vi "Reward Demo (SubVI).vi"(10 "Action":i32, 11 "State":i32) -> (3 "Reward":dbl format="%#_13g")   [LabVIEW 2013]
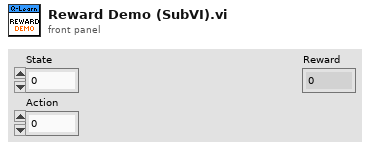
[diagram p1: front panel]
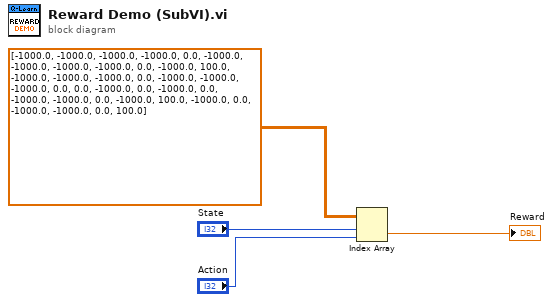
[diagram p0: block diagram]
diagram:
  n1 = Index Array(array=dbl[][] [[-1000.0, -1000.0, -1000.0, -1000.0, 0.0, -1000.0], [-1000.0, -1000.0, -1000.0, 0.0, -1000.0, 100.0], [-1000.0, -1000.0, -1000.0, 0.0, -1000.0, -1000.0], [-1000.0, 0.0, 0.0, -1000.0, 0.0, -1000.0], [0.0, -1000.0, -1000.0, 0.0, -1000.0, 100.0], [-1000.0, 0.0, -1000.0, -1000.0, 0.0, 100.0]], index (row)="State", index (col)="Action") -> (element=→"Reward":dbl)
